vi "targeting.vi"(11 "Degreee Offset":dbl) -> (1 "In Range?":bool, 2 "Right":dbl, 3 "Left":dbl)   [LabVIEW 2020]
uses:
  Framework/Robot Global Data.vi
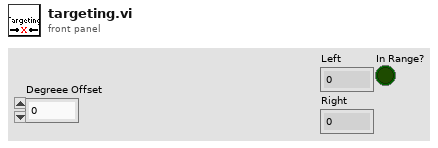
[diagram p1: front panel]
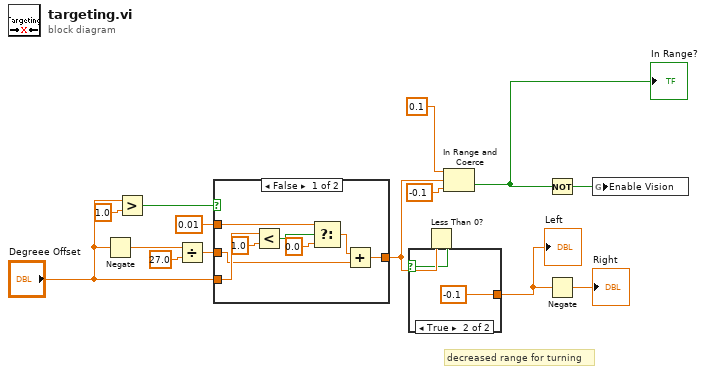
[diagram p0: block diagram]
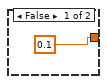
[diagram p2: hidden frame]
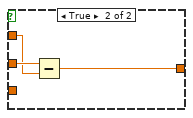
[diagram p3: hidden frame]
diagram:
  # "decreased range for turning"
  n1 = Negate(x="Degreee Offset") -> (-x=w10:dbl)
  n2 = Greater?(x="Degreee Offset", y=1.0) -> (0:w11:bool)
  n3 = Divide(x=w10, y=27.0) -> (x/y=w8:dbl)
  n4 = case shown="False" w11 {
    tunnel: "Degreee Offset" -> [w23 _]
    tunnel: w8 -> [w16 w25]
    tunnel: 0.01 -> [w20 w24]
    tunnel: [w18 w26] -> w3
    frame False {
      n5 = Less?(x=w23, y=1.0) -> (x < y?=w21:bool)
      n6 = Select(t=w20, s=w21, f=0.0) -> (s? t:f=w17:dbl)
      n7 = Add(x=w17, y=w16) -> (x+y=w18:dbl)
    }
    frame True {
      n8 = Subtract(x=w25, y=w24) -> (x-y=w26:dbl)
    }
  }
  n9 = Less Than 0?(x=w3) -> (x < 0?=w2:bool)
  n10 = case shown="True" w2 {
    tunnel: [0.1 -0.1] -> w1
    frame False {
    }
    frame True {
    }
  }
  "Left" <- w1
  n11 = In Range and Coerce(upper limit=0.1, x=w3, lower limit=-0.1) -> (In Range?=w4:bool)  [unwired: 1 out]
  "In Range?" <- w4
  n12 = Not(x=w4) -> (.not. x?=w13:bool)
  n13 = Negate(x=w1) -> (-x=→"Right":dbl)
  n14 = global write "Robot Global Data.vi" "Enable Vision"(w13) -> ()
